vi "Select Box.vi"(8 "error in (no error)":errorcluster, 10 "UI message":string, 11 "Selections available":string[](array[string])) -> (0 "error out":errorcluster, 3 "Selection":string)   [LabVIEW 2019, in "Personalities Tool.lvlib"]
doc: "This VI allows you to create a selector box for the UI."
uses:
  Personalities Tool.lvlib
panel:
  out "Message":string
  in  "Select":bool
  in  "Select":string(combo)
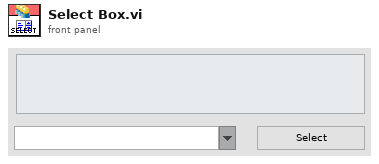
[diagram p1: front panel]
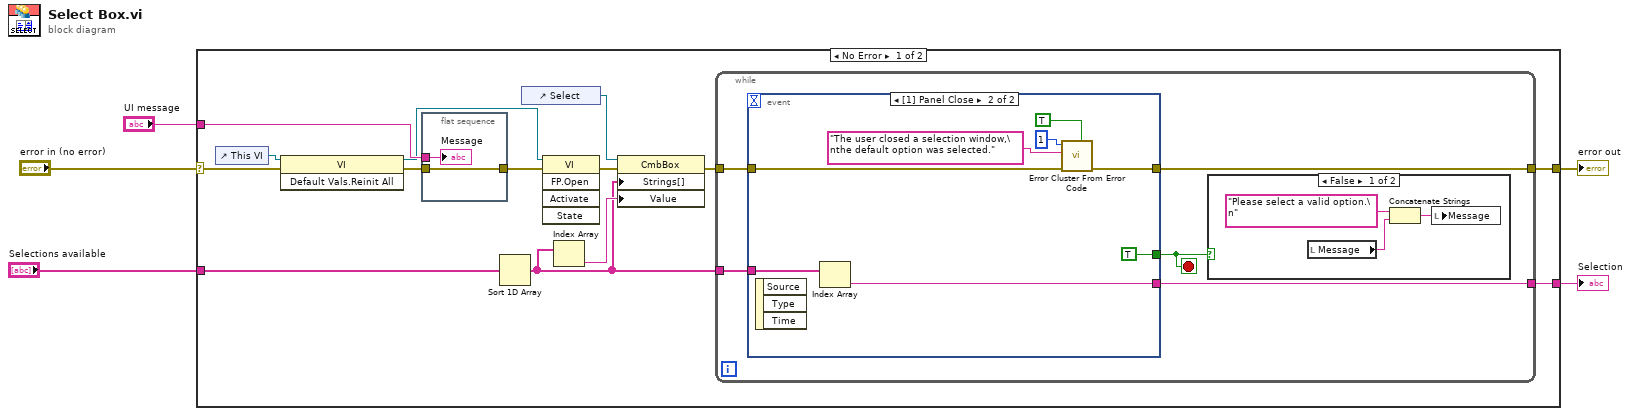
[diagram p0: block diagram]
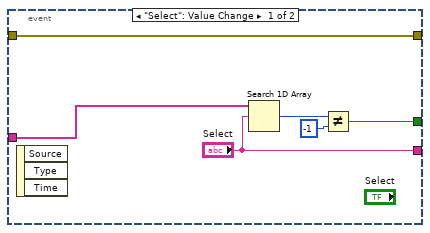
[diagram p3: hidden frame]
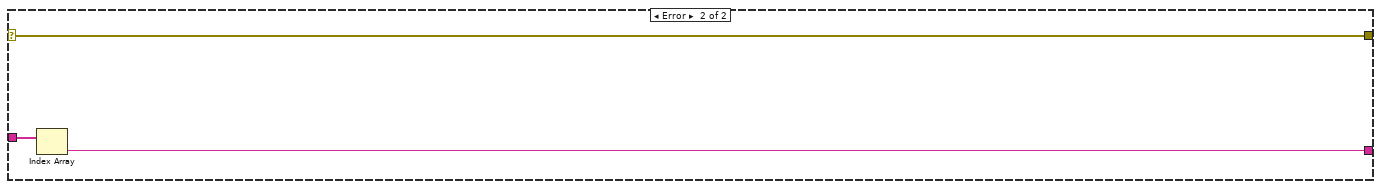
[diagram p4: hidden frame]
diagram:
  n1 = case shown="No Error" "error in (no error)" {
    selector: "error in (no error)" -> [w19 w44]
    tunnel: [w6 w44] -> w4
    tunnel: "Selections available" -> [w8 w46]
    tunnel: [w16 w45] -> w2
    tunnel: "UI message" -> [w14 _]
    frame No Error {
      n2 = control-ref of="This VI"() -> (w13:refnum<vi>)
      n3 = invoke class="VI" method="Default Vals.Reinit All"(reference=w13, error in=w19) -> (reference out=w12:refnum<vi>, error out=w10:errorcluster)  [unwired: 1 in, 1 out]
      n4 = flat-sequence {
        tunnel: w14 -> [w43]
        tunnel: [w42] -> w11
        tunnel: w10 -> [w42]
        frame #0 {
          "Message" <- w43
        }
      }
      n5 = Sort 1D Array(array=w8) -> (sorted array=w7:string[])
      n6 = control-ref of="Select"() -> (w15:refnum<vi>)
      n7 = invoke class="VI" method="FP.Open"(reference=w12, error in=w11) -> (error out=w18:errorcluster)  [unwired: 3 in, 4 out]
      n8 = Index Array(array=w7) -> (element=w9:string)  [unwired: 1 in]
      n9 = property class="CmbBox"(reference=w15, error in=w18, "Strings[]"=w7, "Value"=w9) -> (error out=w17:errorcluster)  [unwired: 1 out]
      n10 = while {
        tunnel: w17 -> [w24]
        tunnel: [w23] -> w16
        tunnel: w7 -> [w22]
        tunnel: [w20] -> w6
        stop <- w21 stop-if-true
        n11 = event shown="[1] Panel Close" {
          selector: _ -> [_ _]
          dyn-events: _ -> [_ _]
          timeout: _ -> [_ _]
          tunnel: w24 -> [w28 w38]
          tunnel: ["Select" w39] -> w23
          tunnel: w22 -> [w33 w40]
          tunnel: [w29 TRUE] -> w21
          tunnel: [w28 w37] -> w20
          event "Select": Value Change {
            n12 = event-data() -> ()  [unwired: 1 in, 3 out]
            n13 = Search 1D Array(1D array=w33, element="Select") -> (index of element=w31:i32)  [unwired: 1 in]
            n14 = Not Equal?(x=w31, y=-1) -> (x != y?=w29:bool)
          }
          event Panel Close {
            n15 = event-data() -> ()  [unwired: 1 in, 3 out]
            n16 = Index Array(array=w40) -> (element=w39:string)  [unwired: 1 in]
            n17 = call <vilib>:"Error Cluster From Error Code.vi"("is warning? (False)"=TRUE, "error in (no error)"=w38, "error message (\"\")"="The user closed a selection window,\nthe default option was selected." ("error message (\"\")"), "error code (0)"=1) -> ("error out"=w37:errorcluster)  [unwired: 5 in]
          }
        }
        n18 = case shown="False" w21 {
          frame False {
            n19 = local read "Message"() -> (w25:string)
            n20 = Concatenate Strings("Please select a valid option.\n" ("Message"), w25) -> (w26:string)
            n21 = local write "Message"(w26) -> ()
          }
          frame True {
          }
        }
      }
    }
    frame Error {
      n22 = Index Array(array=w46) -> (element=w45:string)  [unwired: 1 in]
    }
  }
  "error out" <- w4
  "Selection" <- w2
